vi "Demo1_Subscriber.vi"() -> ()   [LabVIEW 2019]
uses:
  <vilib>/LabVIEW Open Source Project/OpenSerializer/Serializer/Serializer.lvclass
  <vilib>/LabVIEW Open Source Project/MQTT Connection/MQTT_Base/Base Class/MQTT_Base.lvclass/MQTT_Base.ctl
  <vilib>/LabVIEW Open Source Project/MQTT Client/Client class/Client.lvclass/Client.ctl
  <vilib>/LabVIEW Open Source Project/MQTT TCP Connection/MQTT_TCP/Connection/TCPConnection.lvclass
  C:/Program Files (x86)/National Instruments/LabVIEW 2019/vi.lib/LabVIEW Open Source Project/MQTT Connection/MQTT_Connection/Connection/Connection.lvclass
  <vilib>/LabVIEW Open Source Project/MQTT Client/Client class/Client.lvclass
  C:/Program Files (x86)/National Instruments/LabVIEW 2019/vi.lib/LabVIEW Open Source Project/MQTT Connection/MQTT_Base/Base Class/MQTT_Base.lvclass
  <vilib>/LabVIEW Open Source Project/OpenSerializer/Serializer.FlattenedString/Serializer.FlattenedString.lvclass
  C:/Program Files (x86)/National Instruments/LabVIEW 2019/vi.lib/LabVIEW Open Source Project/OpenSerializer/Serializer/Serializer.lvclass
  <vilib>/LabVIEW Open Source Project/MQTT Control Packets/Control Packets/PUBLISH/PUBLISH.lvclass
  <vilib>/LabVIEW Open Source Project/MQTT Connection/MQTT_Base/Base Class/MQTT_Base.lvclass
  <vilib>/LabVIEW Open Source Project/OpenSerializer.Base64/Serializer.Base64.lvclass
  <vilib>/LabVIEW Open Source Project/OpenSerializer JKI JSON/Serializer.JSON.lvclass
panel:
  out "Unsuback":bool
  out "Suback":bool
  in  "Subscribe":bool
  in  "Connection":bool
  in  "Stop Client":bool
  out "Waveform Chart":dbl(graph)
  out "last error":errorcluster
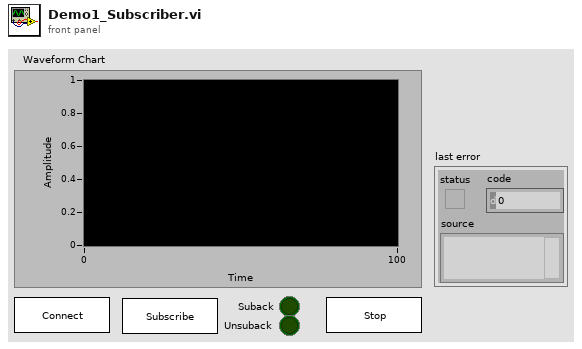
[diagram p1: front panel]
types:
  T1 = typedef "MQTT Client.lvlib/Client.lvclass/Public Events -- cluster.ctl" = cluster{"Connection Status":refnum<user-event>, "Connected":refnum<user-event>, "Application Message":refnum<user-event>}
  T2 = typedef "MQTT Base.lvlib/MQTT_Base.lvclass/Public Events -- cluster.ctl" = cluster{"Stop Event":refnum<user-event>, "Error Event":refnum<user-event>, "Inbound Message":refnum<user-event>}
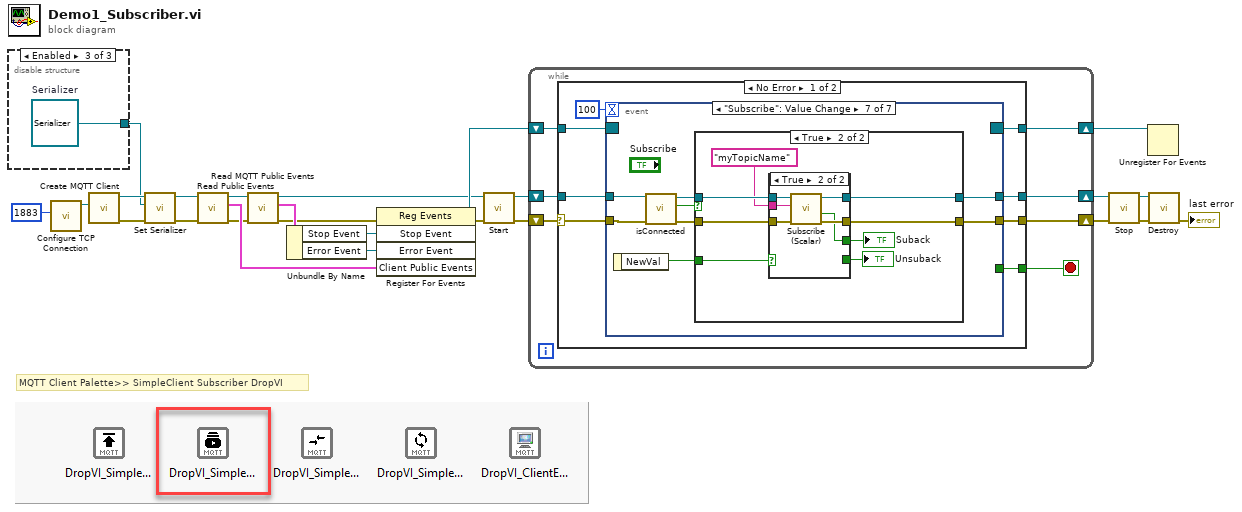
[diagram p0: block diagram]
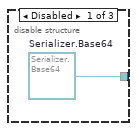
[diagram p2: hidden frame]
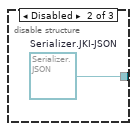
[diagram p3: hidden frame]
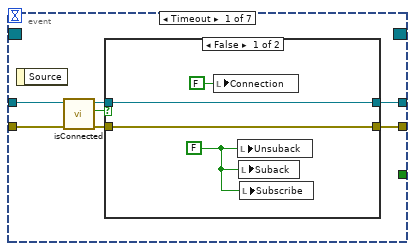
[diagram p4: hidden frame]
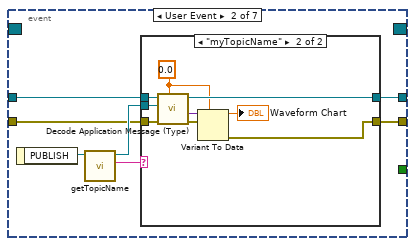
[diagram p6: hidden frame]
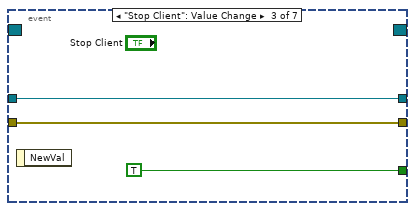
[diagram p8: hidden frame]
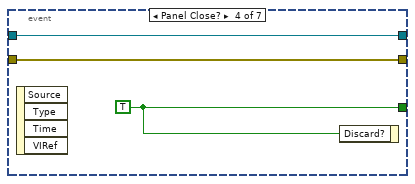
[diagram p9: hidden frame]
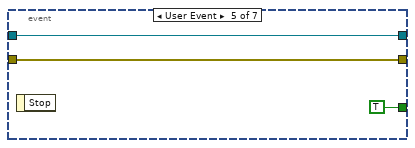
[diagram p10: hidden frame]
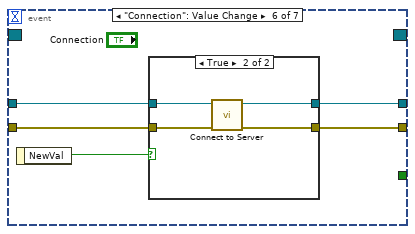
[diagram p11: hidden frame]
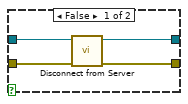
[diagram p12: hidden frame]
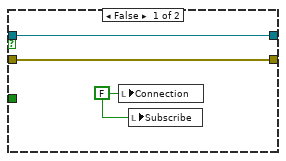
[diagram p13: hidden frame]
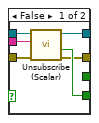
[diagram p14: hidden frame]
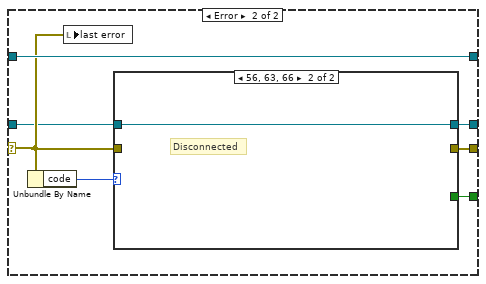
[diagram p15: hidden frame]
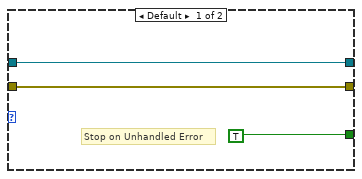
[diagram p16: hidden frame]
diagram:
  # "MQTT Client Palette>> SimpleClient Subscriber DropVI"
  n1 = disable-structure shown="Enabled" {
    disable-tunnel: [w26 w27 w28] -> w1
    frame Disabled {
      w26 = refnum<class "Serializer.Base64.lvclass"> refnum  # Serializer.Base64
    }
    frame Disabled {
      w27 = refnum<class "Serializer.JSON.lvclass"> refnum  # Serializer.JKI-JSON
    }
    frame Enabled {
      w28 = refnum<class "Serializer.lvclass"> refnum  # Serializer
    }
  }
  n2 = call <vilib>:"Configure TCP Connection.vi"("remote port (80)"=u16 1883) -> ("TCPConnection"=w6:refnum<class "TCPConnection.lvclass">)  [unwired: 9 in, 1 out]
  n3 = call <vilib>:"Create MQTT Client.vi"("Connection Configuration"=w6) -> ("error out"=w4:errorcluster, "Client out"=w5:refnum<class "Client.lvclass">)  [unwired: 9 in]
  n4 = call <vilib>:"Set Serializer.vi"("error in (no error)"=w4, "Serializer (default: Flattened String)"=w1, "MQTT_Base"=w5) -> ("error out"=w3:errorcluster, "MQTT_Base out"=w2:refnum<class "Client.lvclass">)  [unwired: 7 in]
  n5 = call <vilib>:"Read Public Events.vi"("error in (no error)"=w3, "Client in"=w2) -> ("error out"=w8:errorcluster, "Client Public Events"=w10:T1, "Client out"=w7:refnum<class "Client.lvclass">)  [unwired: 7 in]
  n6 = call <vilib>:"Read MQTT Public Events.vi"("error in (no error)"=w8, "MQTT_Base in"=w7) -> ("error out"=w9:errorcluster, "MQTT Public Events"=w17:T2, "MQTT_Base out"=w12:refnum<class "Client.lvclass">)  [unwired: 7 in]
  n7 = Unbundle By Name(w17) -> ("Stop Event"=w15:refnum<user-event>, "Error Event"=w16:refnum<user-event>)
  n8 = register-events(error in=w9, w15, w16, w10) -> (reference out=w13:refnum<event-registration>, error out=w11:errorcluster)  [unwired: 1 in]
  n9 = call <vilib>:"Start.vi"("error in (no error)"=w11, "MQTT_Base in"=w12) -> ("error out"=w23:errorcluster, "MQTT_Base out"=w22:refnum<class "Client.lvclass">)  [unwired: 7 in, 1 out]
  n10 = while {
    shift-right: [w34] -> w14
    shift-left: w13 -> [w35]
    shift-right: [w31] -> w19
    shift-left: w22 -> [w32]
    shift-right: [w33] -> w21
    shift-left: w23 -> [w29]
    stop <- w30 stop-if-true
    n11 = case shown="No Error" w29 {
      selector: w29 -> [w36 w131]
      tunnel: w35 -> [w43 w134]
      tunnel: [w42 w134] -> w34
      tunnel: [w41 w129] -> w33
      tunnel: w32 -> [w39 w130]
      tunnel: [w38 w133] -> w31
      tunnel: [w37 w128] -> w30
      frame No Error {
        n12 = event shown="[6] \"Subscribe\": Value Change" {
          selector: w43 -> [_ _ _ _ _ _ _]
          dyn-events: [_ _ _ _ _ _ _] -> w42
          timeout: 100 -> [_ _ _ _ _ _ _]
          tunnel: w36 -> [w46 w60 w76 w78 w83 w84 w102]
          tunnel: [w49 w57 w76 w78 w83 w85 w103] -> w41
          tunnel: [_ _ TRUE w80 TRUE _ _] -> w37
          tunnel: w39 -> [w48 w61 w77 w79 w81 w88 w101]
          tunnel: [w50 w59 w77 w79 w81 w86 w104] -> w38
          event Timeout {
            n13 = event-data() -> ()  [unwired: 1 in, 1 out]
            n14 = call <vilib>:"isConnected.vi"("error in (no error)"=w46, "Client in"=w48) -> ("error out"=w45:errorcluster, "connected"=w44:bool, "Client out"=w47:refnum<class "Client.lvclass">)  [unwired: 7 in]
            n15 = case shown="False" w44 {
              tunnel: [w54 w56] -> w50
              tunnel: [w53 w55] -> w49
              tunnel: w47 -> [w54 w56]
              tunnel: w45 -> [w53 w55]
              frame False {
                w52 = FALSE
                n16 = local write "Connection"(FALSE ("Connection")) -> ()
                n17 = local write "Unsuback"(w52) -> ()
                n18 = local write "Suback"(w52) -> ()
                n19 = local write "Subscribe"(w52) -> ()
              }
              frame True {
              }
            }
          }
          event User Event {
            n20 = event-data() -> ("PUBLISH"=w63:refnum<class "PUBLISH.lvclass">)  [unwired: 1 in]
            n21 = call <vilib>:"getTopicName.vi"("PUBLISH in"=w63) -> ("Topic"=w58:string, "PUBLISH out"=w62:refnum<class "PUBLISH.lvclass">)  [unwired: 8 in, 1 out]
            n22 = case shown="\"myTopicName\"" w58 {
              tunnel: w62 -> [_ w66]
              tunnel: w61 -> [w65 w72]
              tunnel: w60 -> [w64 w70]
              tunnel: [w65 w71] -> w59
              tunnel: [w64 w74] -> w57
              frame Default {
              }
              frame "myTopicName" {
                w68 = 0.0
                n23 = call <vilib>:"Decode Application Message (Type).vi"("Type"=w68, "error in (no error)"=w70, "PUBLISH"=w66, "Client in"=w72) -> ("error out"=w69:errorcluster, "Payload"=w67:variant, "Client out"=w71:refnum<class "Client.lvclass">)  [unwired: 4 in, 1 out]
                n24 = Variant To Data(error in=w69, type=w68, Variant=w67) -> (data=→"Waveform Chart":dbl, error out=w74:errorcluster)
              }
            }
          }
          event "Stop Client": Value Change {
            n25 = event-data() -> ()  [unwired: 1 in, 1 out]
          }
          event Panel Close? {
            w80 = TRUE
            n26 = event-data() -> ()  [unwired: 1 in, 4 out]
            n27 = event-data("Discard?"=w80) -> ()  [unwired: 1 in, 1 out]
          }
          event User Event {
            n28 = event-data() -> ()  [unwired: 1 in, 1 out]
          }
          event "Connection": Value Change {
            n29 = event-data() -> ("NewVal"=w87:bool)  [unwired: 1 in]
            n30 = case shown="True" w87 {
              tunnel: w88 -> [w92 w96]
              tunnel: [w91 w93] -> w86
              tunnel: [w90 w94] -> w85
              tunnel: w84 -> [w89 w95]
              frame False {
                n31 = call <vilib>:"Disconnect from Server.vi"("error in (no error)"=w89, "Client in"=w92) -> ("error out"=w90:errorcluster, "Client out"=w91:refnum<class "Client.lvclass">)  [unwired: 7 in, 1 out]
              }
              frame True {
                n32 = call <vilib>:"Connect to Server.vi"("error in (no error)"=w95, "Client in"=w96) -> ("error out"=w94:errorcluster, "Client out"=w93:refnum<class "Client.lvclass">)  [unwired: 6 in, 2 out]
              }
            }
          }
          event "Subscribe": Value Change {
            n33 = event-data() -> ("NewVal"=w97:bool)  [unwired: 1 in]
            n34 = call <vilib>:"isConnected.vi"("error in (no error)"=w102, "Client in"=w101) -> ("error out"=w99:errorcluster, "connected"=w98:bool, "Client out"=w100:refnum<class "Client.lvclass">)  [unwired: 7 in]
            n35 = case shown="True" w98 {
              tunnel: [w107 w115] -> w104
              tunnel: [w106 w114] -> w103
              tunnel: w100 -> [w107 w113]
              tunnel: w99 -> [w106 w112]
              tunnel: w97 -> [_ w110]
              frame False {
                w105 = FALSE ("Connection")
                n36 = local write "Connection"(w105) -> ()
                n37 = local write "Subscribe"(w105) -> ()
              }
              frame True {
                n38 = case shown="True" w110 {
                  tunnel: [w116 w124] -> w115
                  tunnel: [w117 w123] -> w114
                  tunnel: w113 -> [w121 w127]
                  tunnel: w112 -> [w120 w126]
                  tunnel: "myTopicName" ("Topic Name (empty: Payload name)") -> [w119 w125]
                  tunnel: [_ w122] -> w109
                  tunnel: [w118 _] -> w108
                  frame False {
                    n39 = call <vilib>:"Unsubscribe (Scalar).vi"("error in (no error)"=w120, "Topic Filter"=w119, "Client in"=w121) -> ("error out"=w117:errorcluster, "Ack"=w118:bool, "Client out"=w116:refnum<class "Client.lvclass">)  [unwired: 6 in]
                  }
                  frame True {
                    n40 = call <vilib>:"Subscribe (Scalar).vi"("error in (no error)"=w126, "Topic Filter"=w125, "Client in"=w127) -> ("error out"=w123:errorcluster, "Ack"=w122:bool, "Client out"=w124:refnum<class "Client.lvclass">)  [unwired: 6 in]
                  }
                }
                "Unsuback" <- w108
                "Suback" <- w109
              }
            }
          }
        }
      }
      frame Error {
        n41 = Unbundle By Name(w131) -> ("code"=w132:i32)
        n42 = local write "last error"(w131) -> ()
        n43 = case shown="56, 63, 66" w132 {
          tunnel: w130 -> [w137 w138]
          tunnel: [w137 w138] -> w133
          tunnel: w131 -> [w136 _]
          tunnel: [w136 _] -> w129
          tunnel: [TRUE _] -> w128
          frame Default {
            # "Stop on Unhandled Error"
          }
          frame 56, 63, 66 {
            # "Disconnected"
          }
        }
      }
    }
  }
  n44 = call <vilib>:"Stop.vi"("error in (no error)"=w21, "MQTT_Base in"=w19) -> ("error out"=w20:errorcluster, "MQTT_Base out"=w18:refnum<class "Client.lvclass">)  [unwired: 7 in, 1 out]
  n45 = Unregister For Events(event registration refnum=w14) -> ()  [unwired: 1 in, 1 out]
  n46 = call <vilib>:"Destroy.vi"("error in (no error)"=w20, "MQTT_Base in"=w18) -> ("error out"=→"last error":errorcluster)  [unwired: 8 in, 1 out]
